vi "K_S30_VISA F48.vi"(4 "error in":errorcluster, 7 "Address":u8=250) -> (0 "error out":errorcluster, 2 "SW-Version":string="5.20-3.52", 3 "Information":T1)   [LabVIEW 2012]
panel:
  # "Function 48: initialisation of the device\nV1.0, b.v."
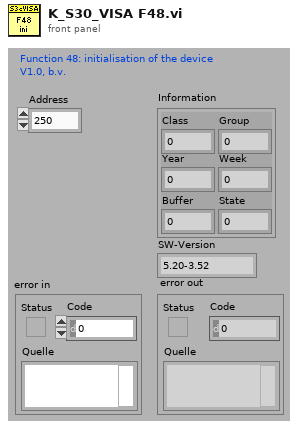
[diagram p1: front panel]
types:
  T1 = cluster{"Class":u8, "Group":u8, "Year":u8, "Week":u8, "Buffer":u8, "State":u8}
  T2 = cluster{"[0]":u8, "[1]":u8, "[2]":u8, "[3]":u8, "[4]":u8, "[5]":u8}
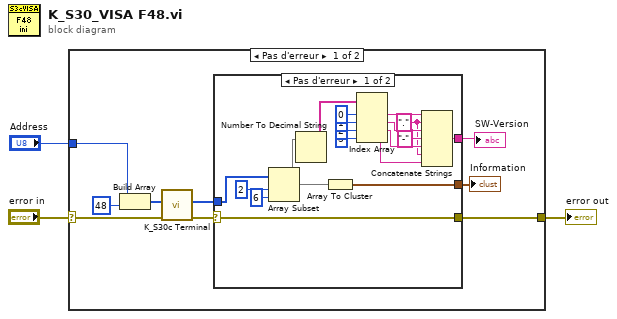
[diagram p0: block diagram]
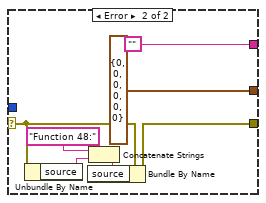
[diagram p2: hidden frame]
diagram:
  n1 = case shown="Pas d'erreur" "error in" {
    selector: "error in" -> [w9 w38]
    tunnel: "Address" -> [w12 _]
    tunnel: [w7 w38] -> w1
    frame No Error {
      n2 = Build Array(w12, u8 48 ("Element")) -> (w10:u8[])
      n3 = call "K_S30c Terminal.vi"("error in"=w9, "request"=w10) -> ("error out"=w8:errorcluster, "response"=w6:u8[])  [unwired: 4 in]
      n4 = case shown="Pas d'erreur" w8 {
        selector: w8 -> [w29 w37]
        tunnel: [w29 w35] -> w7
        tunnel: w6 -> [w21 _]
        tunnel: [w30 cluster{u8, u8, u8, u8, u8, u8} {0, 0, 0, 0, 0, 0} ("response")] -> w5
        tunnel: [w13 ""] -> w4
        frame No Error {
          w18 = "." ("String")
          n5 = Array Subset(array=w21, index=2 ("Index"), length=6 ("Länge")) -> (w26:u8[])
          n6 = Number To Decimal String(number=w26) -> (decimal integer string=w20:string[])  [unwired: 1 in]
          n7 = Array To Cluster(array=w26) -> (cluster=w30:T2)
          n8 = Index Array(array=w20, index #1=0 ("Index"), index #2=1 ("Index"), index #3=2 ("Index"), index #4=3 ("Index")) -> (element #1=w19:string, element #2=w25:string, element #3=w23:string, element #4=w22:string)
          n9 = Concatenate Strings(w19, w18, w25, "-" ("String"), w23, w18, w22) -> (w13:string)
        }
        frame Error {
          n10 = Unbundle By Name(w37) -> ("source"=w32:string)
          n11 = Concatenate Strings("Function 48:" ("String"), w32) -> (w36:string)
          n12 = Bundle By Name(cluster=w37, "source"=w36) -> (w35:errorcluster)
        }
      }
      "SW-Version" <- w4
      "Information" <- w5
    }
    frame Error {
    }
  }
  "error out" <- w1
